vi "Save.vi"(8 "error in (no error)":errorcluster, 11 "Class in":refnum<class "AB_UI_Frmwk_Installer.lvclass">) -> (0 "error out":errorcluster, 2 "build spec name":string, 3 "Class out":refnum<class "AB_UI_Frmwk_Installer.lvclass">)   [LabVIEW 2020, in "AB_UI_Frmwk_Installer.lvclass"]
uses:
  <vilib>/AppBuilder/IB_Classes/Installer/UI/AB_UI_Frmwk_Installer.lvclass
  <vilib>/AppBuilder/IB_Classes/Installer/UI/AB_UI_Frmwk_Installer.lvclass/AB_UI_Frmwk_Installer.ctl
  <vilib>/AppBuilder/IB_Classes/Installer/Installer.lvclass
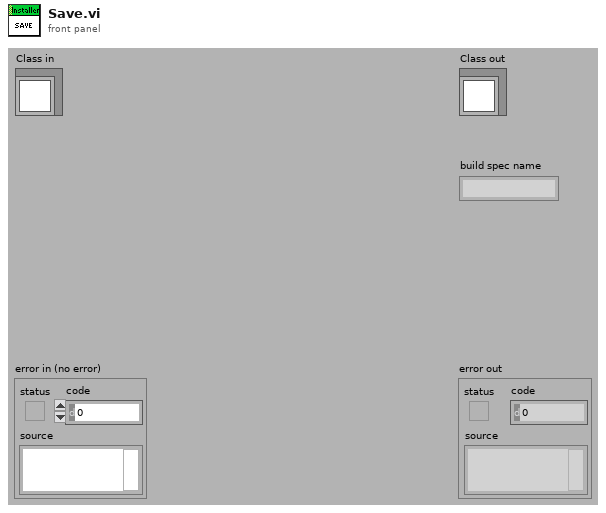
[diagram p1: front panel]
types:
  T1 = typedef "IB_Installer.ctl" = cluster{"Destination":refnum<class "IB_Destination.lvclass">[], "Source":refnum<class "IB_Source.lvclass">[], "buildObject":T2, "defaultDir":string, "platform":string, "author":string, "productName":string, "buildSpecName":string, "hide":bool, "requireLVDevSys":bool, "autoIncrement":bool, "includeError":bool, "readmeID":string, "buildLocation":path, "readmePath":path, "mediaSize":u16, "language":T3, "productVersion":T4, "preview":bool, "programmatic":bool, "progressBarEvents":T5, "userLog_Path":path, "shortcutAddresses":T7[], "EXE_Install Address":string, "EXE_Uninstall Address":string, "additional NIPaths":refnum<class "Dest_NI_NIPath.lvclass">[], "web service itemIDs":string[], "installerName":string}
  T2 = typedef "ItemRef.ctl" = u64
  T3 = typedef "CDK_sTypeDef_Languages.ctl" = u16
  T4 = typedef "CDK_sTypeDef_ProductVersion.ctl" = cluster{"Major":u8, "Minor":u8, "Update":u16}
  T5 = typedef "provcom_ProgressBar_Events.ctl" = cluster{"newJob":refnum<user-event>, "newItem":refnum<user-event>, "errorMsg":T6, "cancel":refnum<user-event>}
  T6 = typedef "mxLvBuildError.ctl" = refnum<user-event>
  T7 = typedef "CDK_sTypeDef_ShortcutAddress.ctl" = cluster{"file":string, "shortcut":string}
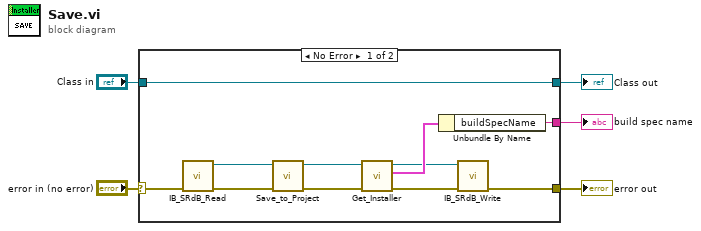
[diagram p0: block diagram]
diagram:
  n1 = case shown="No Error" "error in (no error)" {
    selector: "error in (no error)" -> [w12 w18]
    tunnel: [w7 w18] -> w3
    tunnel: [w16 w17] -> w4
    tunnel: "Class in" -> [w16 w17]
    tunnel: [w15 _] -> w1
    frame No Error {
      n2 = call <resource>:"IB_SRdB_Read.vi"("error in (no error)"=w12) -> ("error out"=w13:errorcluster, "installer out"=w14:refnum<class "Installer.lvclass">)  [unwired: 9 out]
      n3 = call-dynamic "Save_to_Project.vi"("error in (no error)"=w13, "Installer in"=w14) -> ("error out"=w9:errorcluster, "Installer out"=w11:refnum<class "Installer.lvclass">)  [unwired: 8 out]
      n4 = call <vilib>:"Get_Installer.vi"("error in (no error)"=w9, "Installer in"=w11) -> ("error out"=w8:errorcluster, "data"=w10:T1, "Installer out"=w6:refnum<class "Installer.lvclass">)  [unwired: 7 out]
      n5 = Unbundle By Name(w10) -> ("buildSpecName"=w15:string)
      n6 = call <resource>:"IB_SRdB_Write.vi"("error in (no error)"=w8, "installer"=w6) -> ("error out"=w7:errorcluster)  [unwired: 9 out]
    }
    frame Error {
    }
  }
  "error out" <- w3
  "Class out" <- w4
  "build spec name" <- w1
